vi "From ISO8601 String.vi"(11 "ISO-8601":string) -> (2 "error out":errorcluster, 3 "time stamp":timestamp)   [LabVIEW 2020, in "CDM-Config.lvlib"]
doc: "Converts an ISO-8601 formatted timestamp string into a LabVIEW timestamp. ISO-8601 formatted timestamps is the standard used for representing timestamps as a string in this configuration format."
uses:
  CDM-Config.lvlib
  <vilib>/Utility/miscctls.llb/LVDateTimeRec.ctl
  <vilib>/regexp/Match Regular Expression.xnode
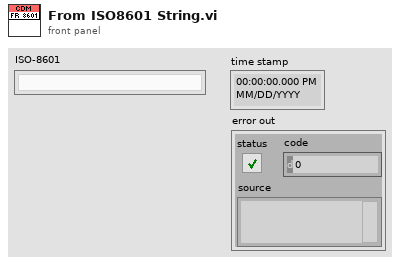
[diagram p1: front panel]
types:
  T1 = typedef "LVDateTimeRec.ctl" = cluster{"fractional second":dbl, "second":i32, "minute":i32, "hour":i32, "day of month":i32, "month":i32, "year":i32, "day of week":i32, "day of year":i32, "DST":i32}
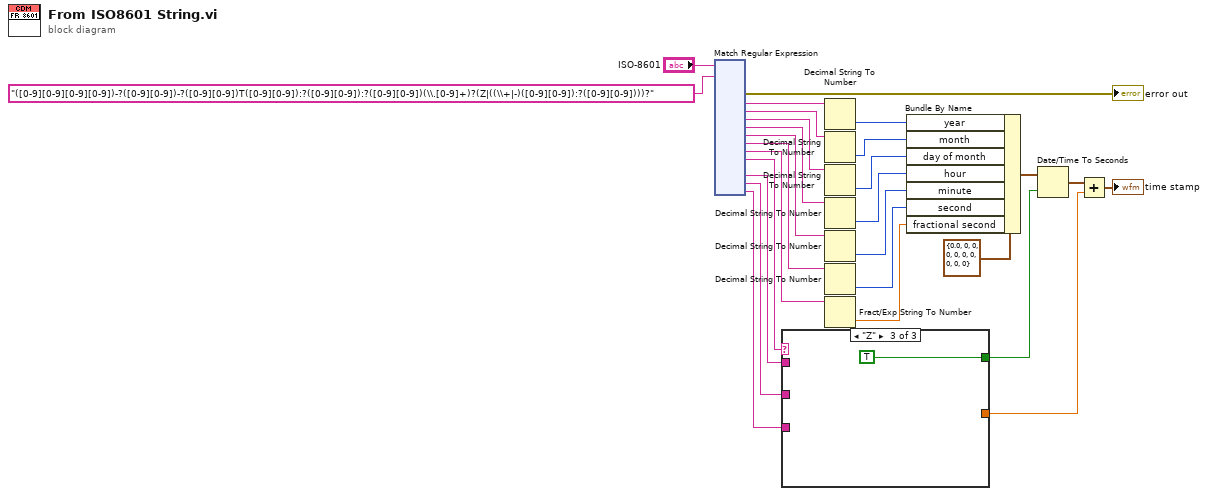
[diagram p0: block diagram]
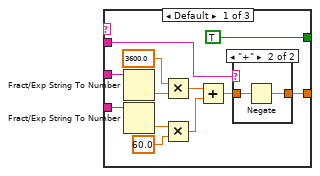
[diagram p2: hidden frame]
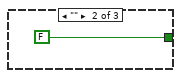
[diagram p4: hidden frame]
diagram:
  n1 = xnode "Match Regular Expression"("input string"="ISO-8601", "regular expression"="([0-9][0-9][0-9][0-9])-?([0-9][0-9])-?([0-9][0-9])T([0-9][0-9]):?([0-9][0-9]):?([0-9][0-9])(\\.[0-9]+)?(Z|((\\+|-)([0-9][0-9]):?([0-9][0-9])))?") -> ("error out"=→"error out":errorcluster, "submatch 1"=w25:string, "submatch 2"=w24:string, "submatch 3"=w15:string, "submatch 4"=w14:string, "submatch 5"=w13:string, "submatch 6"=w12:string, "submatch 7"=w11:string, "submatch 8"=w10:string, "submatch 10"=w9:string, "submatch 11"=w8:string, "submatch 12"=w7:string)  [unwired: 4 in, 5 out]
  n2 = case shown="\"Z\"" w10 {
    tunnel: w9 -> [w29 _ _]
    tunnel: w8 -> [w38 _ _]
    tunnel: w7 -> [w37 _ _]
    tunnel: [TRUE FALSE TRUE] -> w5
    tunnel: [w28 _ _] -> w2
    frame Default {
      n3 = Fract/Exp String To Number(string=w38) -> (number=w36:dbl)  [unwired: 3 in, 1 out]
      n4 = Fract/Exp String To Number(string=w37) -> (number=w35:dbl)  [unwired: 3 in, 1 out]
      n5 = Multiply(x=3600.0 ("y"), y=w36) -> (x*y=w32:dbl)
      n6 = Multiply(x=w35, y=60.0) -> (x*y=w31:dbl)
      n7 = Add(x=w32, y=w31) -> (x+y=w30:dbl)
      n8 = case shown="\"+\"" w29 {
        tunnel: w30 -> [w40 w42]
        tunnel: [w40 w41] -> w28
        frame Default {
        }
        frame "+" {
          n9 = Negate(x=w42) -> (-x=w41:dbl)
        }
      }
    }
    frame "" {
    }
    frame "Z" {
    }
  }
  n10 = Decimal String To Number(string=w25) -> (number=w22:i32)  [unwired: 2 in, 1 out]
  n11 = Decimal String To Number(string=w24) -> (number=w21:i32)  [unwired: 2 in, 1 out]
  n12 = Decimal String To Number(string=w15) -> (number=w20:i32)  [unwired: 2 in, 1 out]
  n13 = Decimal String To Number(string=w14) -> (number=w19:i32)  [unwired: 2 in, 1 out]
  n14 = Decimal String To Number(string=w13) -> (number=w18:i32)  [unwired: 2 in, 1 out]
  n15 = Decimal String To Number(string=w12) -> (number=w17:i32)  [unwired: 2 in, 1 out]
  n16 = Fract/Exp String To Number(string=w11) -> (number=w16:dbl)  [unwired: 3 in, 1 out]
  n17 = Bundle By Name(cluster=T1 {"fractional second"=0.0, "second"=0, "minute"=0, "hour"=0, "day of month"=0, "month"=0, "year"=0, "day of week"=0, "day of year"=0, "DST"=0} ("date time rec"), "year"=w22, "month"=w21, "day of month"=w20, "hour"=w19, "minute"=w18, "second"=w17, "fractional second"=w16) -> (w6:T1)
  n18 = Date/Time To Seconds(1:w5, 2:w6) -> (0:w4:timestamp)
  n19 = Add(x=w4, y=w2) -> (x+y=→"time stamp":timestamp)
